vi "YKMW100 Determine Power Relay Status.vi"(8 "Error In":errorcluster, 11 "Full Module List":string[](array[string])) -> (0 "Error Out":errorcluster, 2 "DO Card Detected for Module 5":bool, 3 "Module 4 Relay Status":T1)   [LabVIEW 2020]
uses:
  Trunk/Hybrid Water Heater/Custom Instrument Control/MW100/Type Definitions/HEWH Module 4 Relay Status.ctl
  <vilib>/Utility/error.llb/whitespace.ctl
panel:
  # "Need to add PRAT and RLT Relay Status"
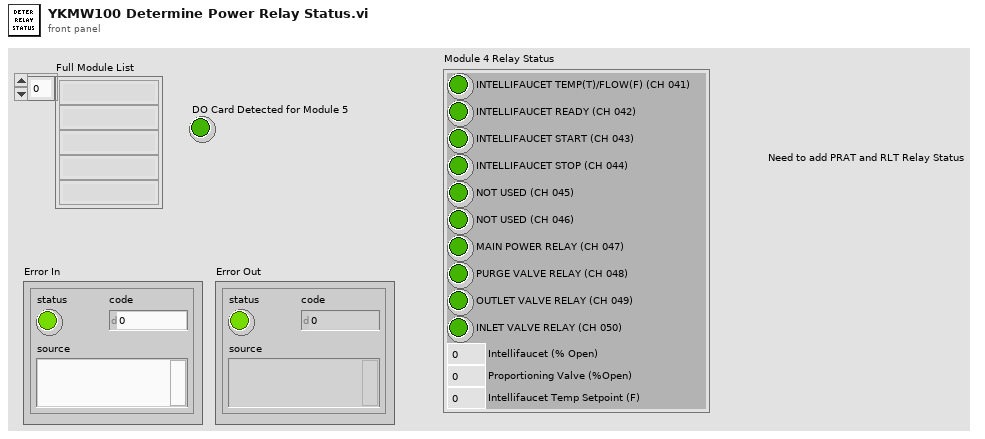
[diagram p1: front panel]
types:
  T1 = typedef "HEWH Module 4 Relay Status.ctl" = cluster{"INTELLIFAUCET TEMP(T)/FLOW(F) (CH 041)":bool, "INTELLIFAUCET READY (CH 042)":bool, "INTELLIFAUCET START (CH 043)":bool, "INTELLIFAUCET STOP (CH 044)":bool, "MAIN POWER RELAY (CH 047)":bool, "NOT USED (CH 045)":bool, "NOT USED (CH 046)":bool, "PURGE VALVE RELAY (CH 048)":bool, "OUTLET VALVE RELAY (CH 049)":bool, "INLET VALVE RELAY (CH 050)":bool, "Intellifaucet (% Open)":dbl, "Proportioning Valve (%Open)":dbl, "Intellifaucet Temp Setpoint (F)":dbl}
  T2 = typedef "whitespace.ctl" = u16
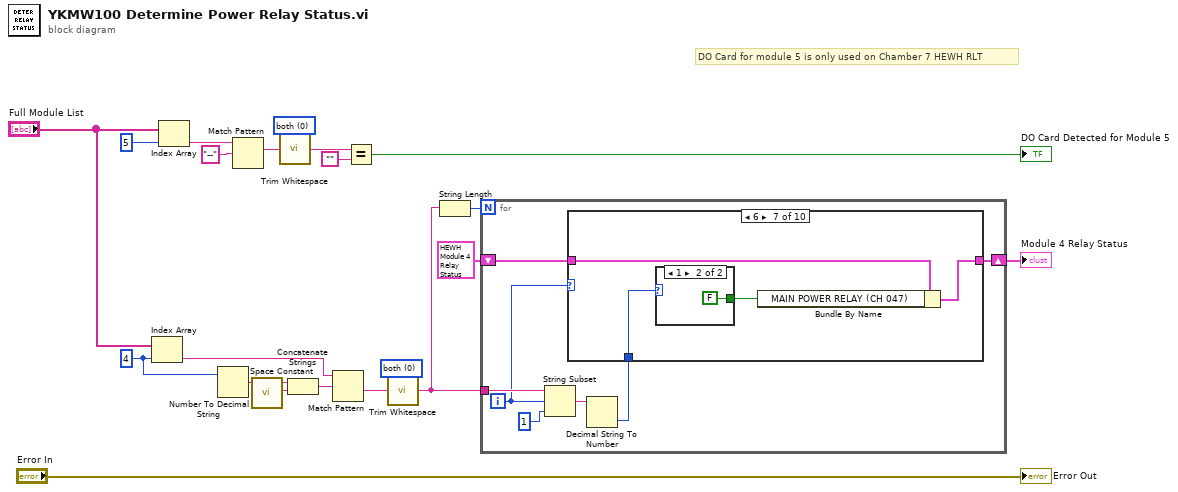
[diagram p0: block diagram]
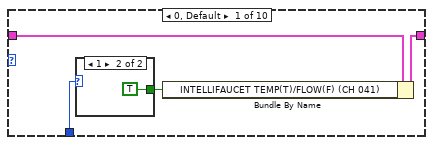
[diagram p2: hidden frame]
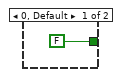
[diagram p3: hidden frame]
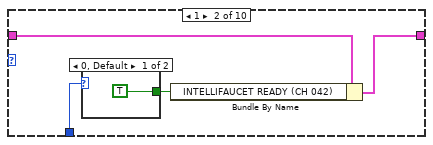
[diagram p4: hidden frame]
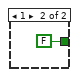
[diagram p5: hidden frame]
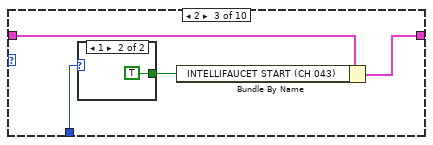
[diagram p6: hidden frame]
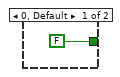
[diagram p7: hidden frame]
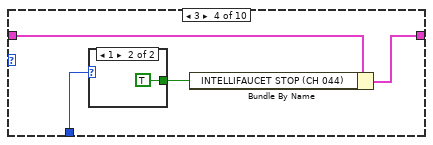
[diagram p8: hidden frame]
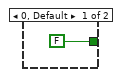
[diagram p9: hidden frame]
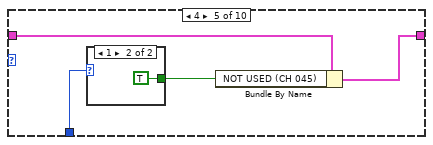
[diagram p10: hidden frame]
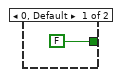
[diagram p11: hidden frame]
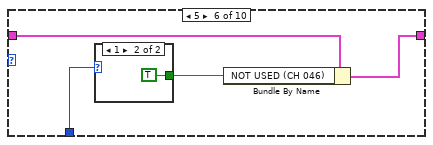
[diagram p12: hidden frame]
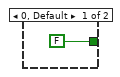
[diagram p13: hidden frame]
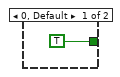
[diagram p14: hidden frame]
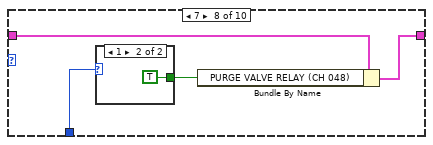
[diagram p15: hidden frame]
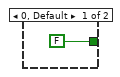
[diagram p16: hidden frame]
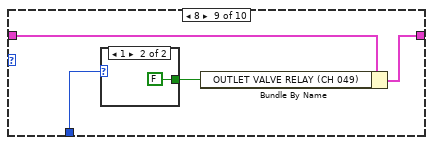
[diagram p17: hidden frame]
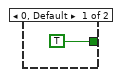
[diagram p18: hidden frame]
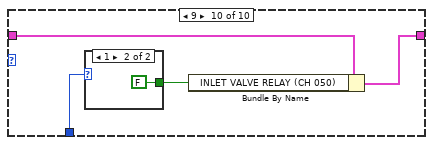
[diagram p19: hidden frame]
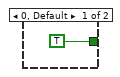
[diagram p20: hidden frame]
diagram:
  w1 = 4 ("Module Number")
  w9 = T2 0 items=["both", "start of string", "end of string"] ("location (both)")
  w16 = T2 0 items=["both", "start of string", "end of string"] ("location (both)")
  # "DO Card for module 5 is only used on Chamber 7 HEWH RLT"
  n1 = Index Array(array="Full Module List", index=w1) -> (element=w14:string)
  n2 = Index Array(array="Full Module List", index=5) -> (element=w7:string)
  n3 = Number To Decimal String(number=w1) -> (decimal integer string=w19:string)  [unwired: 1 in]
  n4 = Match Pattern(string=w7, regular expression="--") -> (match substring=w11:string)  [unwired: 1 in, 3 out]
  n5 = call <vilib>:"Space Constant.vi"() -> ("String"=w20:string)
  n6 = call <vilib>:"Trim Whitespace.vi"("string"=w11, "location (both)"=w9) -> ("trimmed string"=w13:string)
  n7 = Concatenate Strings(w19, w20) -> (w21:string)
  n8 = Match Pattern(string=w14, regular expression=w21) -> (after substring=w15:string)  [unwired: 1 in, 3 out]
  n9 = Equal?(x=w13, y="") -> (x = y?=→"DO Card Detected for Module 5":bool)
  n10 = call <vilib>:"Trim Whitespace.vi"("string"=w15, "location (both)"=w16) -> ("trimmed string"=w18:string)
  n11 = String Length(string=w18) -> (length=w17:i32)
  n12 = for {
    N: w17 -> [_]
    tunnel: w18 -> [w27]
    shift-right: [w23] -> w2
    shift-left: T1 {"INTELLIFAUCET TEMP(T)/FLOW(F) (CH 041)"=FALSE, "INTELLIFAUCET READY (CH 042)"=FALSE, "INTELLIFAUCET START (CH 043)"=FALSE, "INTELLIFAUCET STOP (CH 044)"=FALSE, "MAIN POWER RELAY (CH 047)"=FALSE, "NOT USED (CH 045)"=FALSE, "NOT USED (CH 046)"=FALSE, "PURGE VALVE RELAY (CH 048)"=FALSE, "OUTLET VALVE RELAY (CH 049)"=FALSE, "INLET VALVE RELAY (CH 050)"=FALSE, "Intellifaucet (% Open)"=0.0, "Proportioning Valve (%Open)"=0.0, "Intellifaucet Temp Setpoint (F)"=0.0} ("Module 4 Relay Status") -> [w24]
    i -> [w25]
    n13 = String Subset(string=w27, offset (0)=w25, length (rest)=1 ("length (rest)")) -> (substring=w26:string)
    n14 = Decimal String To Number(string=w26) -> (number=w22:i32)  [unwired: 2 in, 1 out]
    n15 = case shown="6" w25 {
      tunnel: w24 -> [w32 w36 w42 w49 w55 w61 w67 w72 w79 w84]
      tunnel: [w31 w37 w43 w48 w54 w60 w66 w71 w78 w83] -> w23
      tunnel: w22 -> [w30 w35 w41 w47 w53 w59 w65 w73 w77 w85]
      frame 0, Default {
        n16 = case shown="1" w30 {
          tunnel: [FALSE TRUE] -> w29
          frame 0, Default {
          }
          frame 1 {
          }
        }
        n17 = Bundle By Name(cluster=w32, "INTELLIFAUCET TEMP(T)/FLOW(F) (CH 041)"=w29) -> (w31:T1)
      }
      frame 1 {
        n18 = case shown="0, Default" w35 {
          tunnel: [TRUE FALSE] -> w38
          frame 0, Default {
          }
          frame 1 {
          }
        }
        n19 = Bundle By Name(cluster=w36, "INTELLIFAUCET READY (CH 042)"=w38) -> (w37:T1)
      }
      frame 2 {
        n20 = case shown="1" w41 {
          tunnel: [FALSE TRUE] -> w44
          frame 0, Default {
          }
          frame 1 {
          }
        }
        n21 = Bundle By Name(cluster=w42, "INTELLIFAUCET START (CH 043)"=w44) -> (w43:T1)
      }
      frame 3 {
        n22 = case shown="1" w47 {
          tunnel: [FALSE TRUE] -> w50
          frame 0, Default {
          }
          frame 1 {
          }
        }
        n23 = Bundle By Name(cluster=w49, "INTELLIFAUCET STOP (CH 044)"=w50) -> (w48:T1)
      }
      frame 4 {
        n24 = case shown="1" w53 {
          tunnel: [FALSE TRUE] -> w56
          frame 0, Default {
          }
          frame 1 {
          }
        }
        n25 = Bundle By Name(cluster=w55, "NOT USED (CH 045)"=w56) -> (w54:T1)
      }
      frame 5 {
        n26 = case shown="1" w59 {
          tunnel: [FALSE TRUE] -> w62
          frame 0, Default {
          }
          frame 1 {
          }
        }
        n27 = Bundle By Name(cluster=w61, "NOT USED (CH 046)"=w62) -> (w60:T1)
      }
      frame 6 {
        n28 = case shown="1" w65 {
          tunnel: [TRUE FALSE] -> w68
          frame 0, Default {
          }
          frame 1 {
          }
        }
        n29 = Bundle By Name(cluster=w67, "MAIN POWER RELAY (CH 047)"=w68) -> (w66:T1)
      }
      frame 7 {
        n30 = case shown="1" w73 {
          tunnel: [FALSE TRUE] -> w74
          frame 0, Default {
          }
          frame 1 {
          }
        }
        n31 = Bundle By Name(cluster=w72, "PURGE VALVE RELAY (CH 048)"=w74) -> (w71:T1)
      }
      frame 8 {
        n32 = case shown="1" w77 {
          tunnel: [TRUE FALSE] -> w80
          frame 0, Default {
          }
          frame 1 {
          }
        }
        n33 = Bundle By Name(cluster=w79, "OUTLET VALVE RELAY (CH 049)"=w80) -> (w78:T1)
      }
      frame 9 {
        n34 = case shown="1" w85 {
          tunnel: [TRUE FALSE] -> w86
          frame 0, Default {
          }
          frame 1 {
          }
        }
        n35 = Bundle By Name(cluster=w84, "INLET VALVE RELAY (CH 050)"=w86) -> (w83:T1)
      }
    }
  }
  "Module 4 Relay Status" <- w2
  "Error Out" <- "Error In"
